vi "ConnorsCode.vi"() -> ()   [LabVIEW 2020]
uses:
  Subs/ColorText/Code.xctl
  Subs/Console XCtrl/Console_Xctrl.xctl
panel:
  in  "New File":bool
  in  "Py Files":i32(listbox)
  in  "Python Files":path
  in  "Code":string(xcontrol)="import os\n\nfor i in range(10):\n     print(i)\n"
  in  "Files":bool
  in  "Stop":bool
  in  "Run":bool
  out "REPL":string(xcontrol)
  in  "Help files":u16(ring) items=["Battery.py", "Buttons.py", "Display.py", "Image.py", "LED.py", "Motion.py", "Motor.py", "Sound.py"]
  out "Help Code":string(xcontrol)="import os\n\nfor i in range(10):\n     print(i)\n"
  # "Connor's Code"
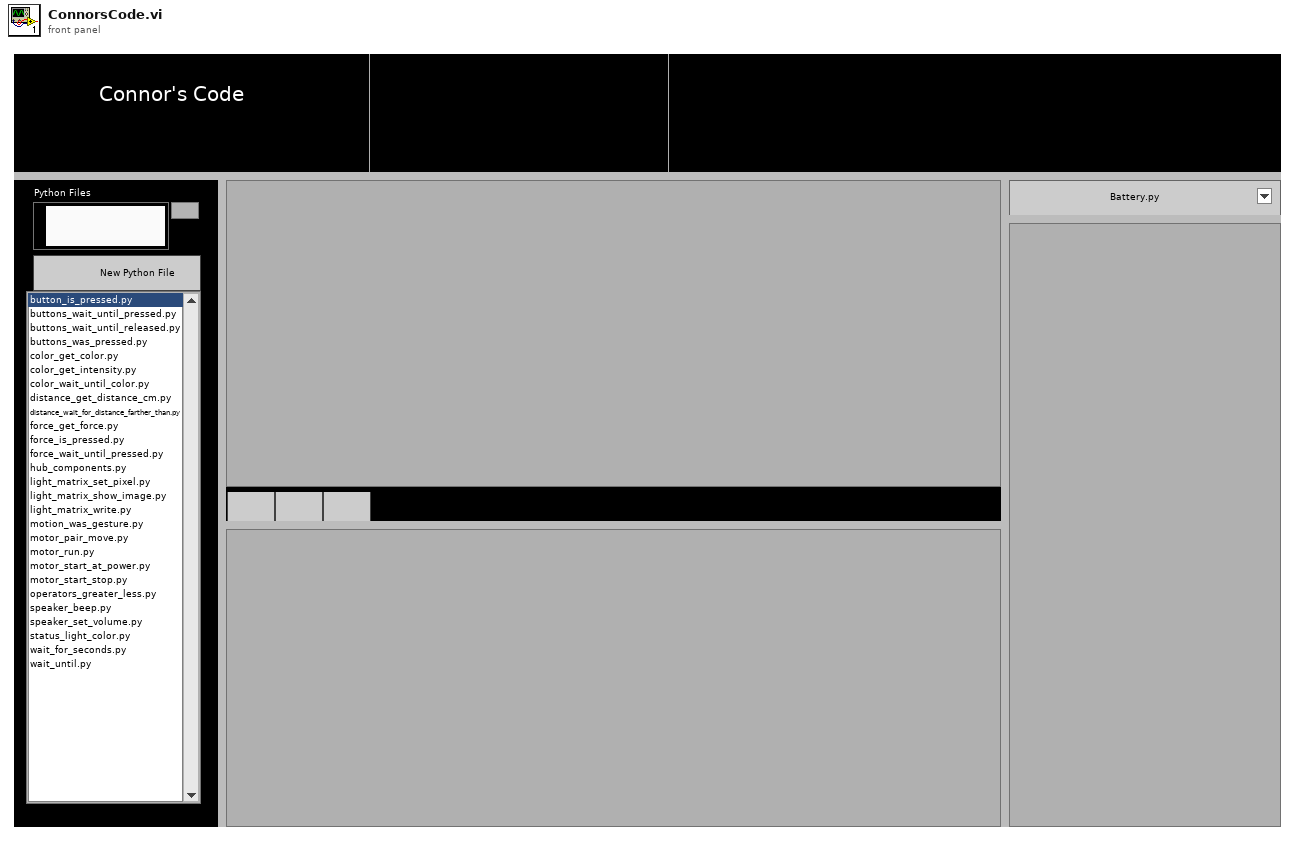
[diagram p1: front panel]
types:
  T1 = cluster{"Quote":u32, "Comment":u32, "Python":u32, "Text":u32, "Triple Quote":u32, "function":u32, "Line numbers":u32, "REPL Err":u32, "REPL Text":u32, "REPL Text 2":u32, "REPL Text 3":u32}
  T2 = typedef "eventvkey.ctl" = enum16{"ASCII", "Enter", "Return", "Shift", "Ctrl", "Alt", "Cmd", "Opt", "Caps", "NumLock", "Clear", "Break", "Up", "Down", "Left", "Right", "Insert", "Delete", "Home", "End", "PageUp", "PageDown", "Escape", "Help", "Pause", "ScrollLock", "F1", "F2", "F3", "F4", "F5", "F6", "F7", "F8", "F9", "F10", "F11", "F12", "F13", "F14", "F15", "F16", "F17", "F18", "F19", "F20", "F21", "F22", "F23", "F24", "Play", "VolumeUp", "VolumeDown", "Mute", "Two Byte Char"}
  T3 = cluster{"Shift":bool, "Ctrl":bool, "Alt":bool, "Cmd":bool, "Opt":bool}
  T4 = cluster{"Char":i16, "VKey":T2, "PlatMods":cluster{"Shift":bool, "Ctrl":bool, "Alt":bool, "Cmd":bool, "Opt":bool}}
  T5 = enum8{"Enabled", "Disabled", "Disabled and Grayed Out"}
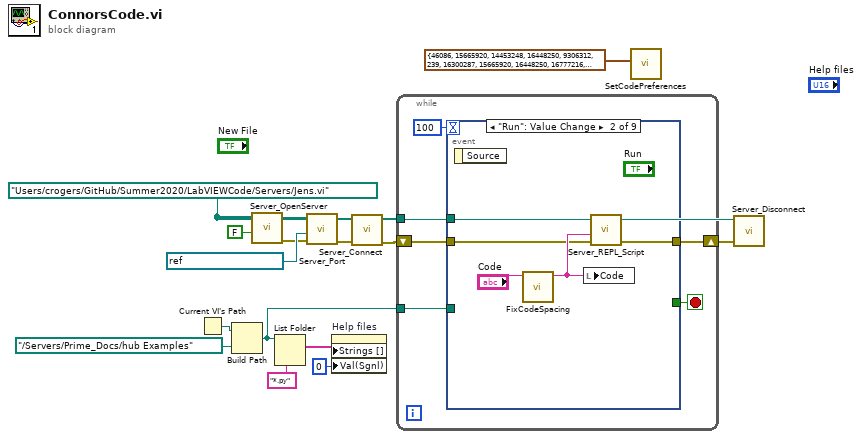
[diagram p0: block diagram]
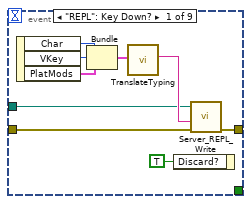
[diagram p2: hidden frame]
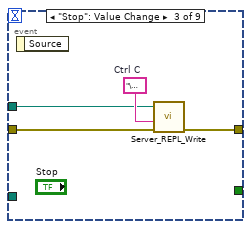
[diagram p3: hidden frame]
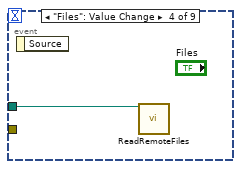
[diagram p4: hidden frame]
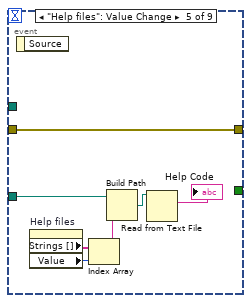
[diagram p5: hidden frame]
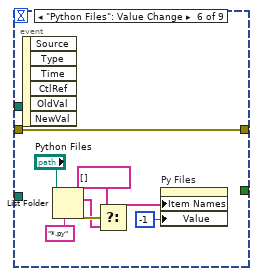
[diagram p6: hidden frame]
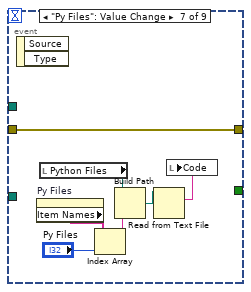
[diagram p7: hidden frame]
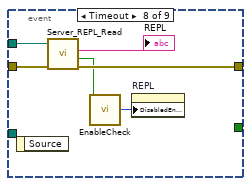
[diagram p8: hidden frame]
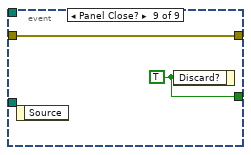
[diagram p9: hidden frame]
diagram:
  w7 = path "/Users/crogers/GitHub/Summer2020/LabVIEWCode/Servers/Jens.vi" ("Server")
  n1 = Current VI's Path() -> (path=w6:path)
  n2 = Build Path(base path=w6, name or relative path=path "../Servers/Prime_Docs/hub Examples") -> (appended path=w2:path)
  n3 = call "Server_OpenServer.vi"("Wait for connection?"=FALSE, "Server"=w7) -> ("error out"=w11:errorcluster)  [unwired: 9 in]
  n4 = List Folder(path=w2, pattern="*.py") -> (filenames=w3:string[])  [unwired: 2 in, 3 out]
  n5 = call "Server_Port.vi"("error in (no error)"=w11, "Port"=refnum<visa-resource-name> "ASRL102::INSTR", "Server"=w7) -> ("error out"=w10:errorcluster)  [unwired: 8 in]
  n6 = property on="Help files" class="Ring (strict)"("Strings []"=w3, "Val(Sgnl)"=0) -> ()  [unwired: 2 in, 2 out]
  n7 = call "Server_Connect.vi"("error in (no error)"=w10, "Server"=w7) -> ("error out"=w9:errorcluster)  [unwired: 9 in]
  n8 = while {
    tunnel: w7 -> [w18]
    shift-right: [w19] -> w8
    shift-left: w9 -> [w20]
    tunnel: w2 -> [w15]
    stop <- w16 stop-if-true
    n9 = event shown="[1] \"Run\": Value Change" {
      selector: _ -> [_ _ _ _ _ _ _ _ _]
      dyn-events: _ -> [_ _ _ _ _ _ _ _ _]
      timeout: 100 -> [_ _ _ _ _ _ _ _ _]
      tunnel: w20 -> [w26 w32 w37 _ w40 w52 w61 w66 w68]
      tunnel: [w25 w31 w36 _ w40 w52 w61 w64 w68] -> w19
      tunnel: w18 -> [w21 w30 w35 w39 _ _ _ w67 _]
      tunnel: [_ _ _ _ _ _ _ _ w69] -> w16
      tunnel: w15 -> [_ _ _ _ w44 _ _ _ _]
      event "REPL": Key Down? {
        n10 = event-data() -> ("Char"=w23:i16, "VKey"=w24:T2, "PlatMods"=w22:T3)  [unwired: 1 in]
        n11 = Bundle("Char"=w23, "VKey"=w24, "PlatMods"=w22) -> (w28:T4)  [unwired: 1 in]
        n12 = call "TranslateTyping.vi"("Cluster"=w28) -> ("key"=w29:string)  [unwired: 10 in]
        n13 = event-data("Discard?"=TRUE) -> ()  [unwired: 1 in, 1 out]
        n14 = call "Server_REPL_Write.vi"("error in (no error)"=w26, "Code"=w29, "Server"=w21) -> ("error out"=w25:errorcluster)  [unwired: 8 in]
      }
      event "Run": Value Change {
        n15 = event-data() -> ()  [unwired: 1 in, 1 out]
        n16 = call "FixCodeSpacing.vi"("Code"="Code") -> ("Cleaned"=w34:string)  [unwired: 10 in]
        n17 = local write "Code"(w34) -> ()
        n18 = call "Server_REPL_Script.vi"("error in (no error)"=w32, "Code"=w34, "Server"=w30) -> ("error out"=w31:errorcluster)  [unwired: 8 in]
      }
      event "Stop": Value Change {
        w38 = "\u0003"  # Ctrl C
        n19 = event-data() -> ()  [unwired: 1 in, 1 out]
        n20 = call "Server_REPL_Write.vi"("error in (no error)"=w37, "Code"=w38, "Server"=w35) -> ("error out"=w36:errorcluster)  [unwired: 8 in]
      }
      event "Files": Value Change {
        n21 = event-data() -> ()  [unwired: 1 in, 1 out]
        n22 = call "ReadRemoteFiles.vi"("Server"=w39) -> ()  [unwired: 11 in]
      }
      event "Help files": Value Change {
        n23 = event-data() -> ()  [unwired: 1 in, 1 out]
        n24 = property on="Help files" class="Ring (strict)"() -> ("Strings []"=w46:string[], "Value"=w45:u16)  [unwired: 2 in, 2 out]
        n25 = Index Array(array=w46, index=w45) -> (element=w43:string)
        n26 = Build Path(base path=w44, name or relative path=w43) -> (appended path=w42:path)
        n27 = Read from Text File(file (use dialog)=w42) -> (text=→"Help Code":string)  [unwired: 3 in, 3 out]
      }
      event "Python Files": Value Change {
        n28 = event-data() -> ()  [unwired: 1 in, 6 out]
        n29 = List Folder(path="Python Files", pattern="*.py") -> (filenames=w49:string[], error out=w50:errorcluster)  [unwired: 2 in, 2 out]
        n30 = Select(t=string[] [], s=w50, f=w49) -> (s? t:f=w48:string[])
        n31 = property on="Py Files" class="LstBox (strict)"("Item Names"=w48, "Value"=-1) -> ()  [unwired: 2 in, 2 out]
      }
      event "Py Files": Value Change {
        n32 = event-data() -> ()  [unwired: 1 in, 2 out]
        n33 = property on="Py Files" class="LstBox (strict)"() -> ("Item Names"=w59:string[])  [unwired: 2 in, 2 out]
        n34 = local read "Python Files"() -> (w57:path)
        n35 = Index Array(array=w59, index="Py Files") -> (element=w58:string)
        n36 = Build Path(base path=w57, name or relative path=w58) -> (appended path=w56:path)
        n37 = Read from Text File(file (use dialog)=w56) -> (text=w55:string)  [unwired: 3 in, 3 out]
        n38 = local write "Code"(w55) -> ()
      }
      event Timeout {
        n39 = event-data() -> ()  [unwired: 1 in, 1 out]
        n40 = call "Server_REPL_Read.vi"("error in (no error)"=w66, "Server"=w67) -> ("error out"=w64:errorcluster, "Running?"=w63:bool, "REPL"=→"REPL":string)  [unwired: 7 in]
        n41 = call "EnableCheck.vi"("Enable?"=w63) -> ("Enum"=w62:T5)
        n42 = property on="REPL" class="Console_Xctrl (strict)"("DisabledEnum"=w62) -> ()  [unwired: 2 in, 2 out]
      }
      event Panel Close? {
        w69 = TRUE ("Discard?")
        n43 = event-data() -> ()  [unwired: 1 in, 1 out]
        n44 = event-data("Discard?"=w69) -> ()  [unwired: 1 in, 1 out]
      }
    }
  }
  n45 = call "SetCodePreferences.vi"("Color choices"=T1 {"Quote"=46086, "Comment"=15665920, "Python"=14453248, "Text"=16448250, "Triple Quote"=9306312, "function"=239, "Line numbers"=16300287, "REPL Err"=15665920, "REPL Text"=16448250, "REPL Text 2"=16777216, "REPL Text 3"=16777216}) -> ()  [unwired: 11 in]
  n46 = call "Server_Disconnect.vi"("error in (no error)"=w8, "Server"=w7) -> ()  [unwired: 9 in, 1 out]
